vi "FGV_PSP - Mercury Remote.vi"(4 "error in":errorcluster, 6 "Function":enum16{"write", "read"}(ring), 7 "Remote":bool) -> (0 "error out":errorcluster, 3 "Remote":bool)   [LabVIEW 2016, in "Instrument.OxfordVRM.lvclass"]
uses:
  Instrument.OxfordVRM.lvclass
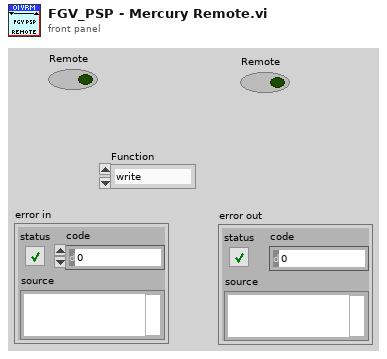
[diagram p1: front panel]
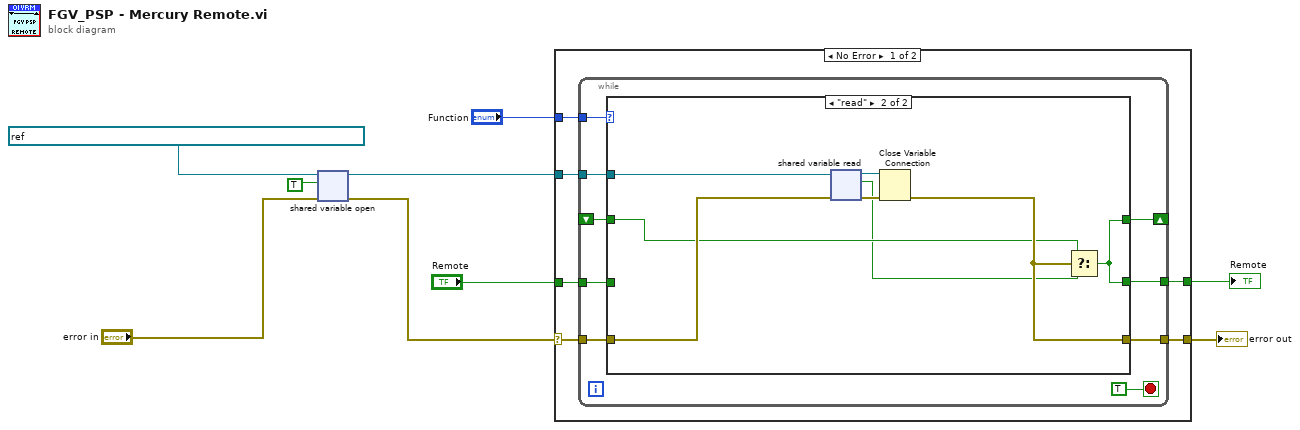
[diagram p0: block diagram]
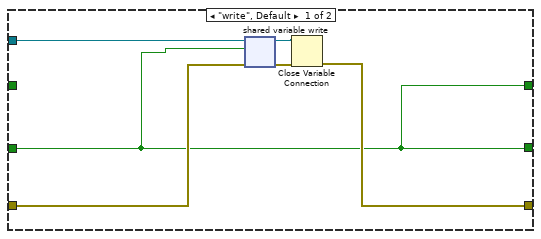
[diagram p2: hidden frame]
diagram:
  n1 = shared-variable-open(refnum<k21> "ni.var.psp://localhost/1820/Mercury_Remote" ("shared variable refnum in"), "error in", TRUE) -> (w7:refnum<k21>, w6:errorcluster)  [unwired: 1 in]
  n2 = case shown="No Error" w6 {
    selector: w6 -> [w15 w40]
    tunnel: [w14 w40] -> w9
    tunnel: [w13 w39] -> w1
    tunnel: "Function" -> [w12 _]
    tunnel: w7 -> [w11 _]
    tunnel: "Remote" -> [w10 w39]
    frame No Error {
      n3 = while {
        shift-right: [w19] -> _
        shift-left: _ -> [w18]
        tunnel: w15 -> [w23]
        tunnel: [w22] -> w14
        tunnel: [w21] -> w13
        tunnel: w12 -> [w20]
        tunnel: w11 -> [w17]
        tunnel: w10 -> [w16]
        stop <- TRUE stop-if-true
        n4 = case shown="\"read\"" w20 {
          tunnel: w23 -> [w29 w36]
          tunnel: [w30 w35] -> w22
          tunnel: [w25 w38] -> w21
          tunnel: [w25 w38] -> w19
          tunnel: w18 -> [_ w34]
          tunnel: w17 -> [w28 w37]
          tunnel: w16 -> [w25 _]
          frame "write", Default {
            n5 = shared-variable-write(w28, w29, w25) -> (w26:refnum<k21>, w27:errorcluster)
            n6 = Close Variable Connection(8:w27, 11:w26) -> (0:w30:errorcluster)
          }
          frame "read" {
            n7 = shared-variable-read(w37, w36) -> (w33:refnum<k21>, w32:errorcluster, w31:bool)  [unwired: 1 out]
            n8 = Close Variable Connection(8:w32, 11:w33) -> (0:w35:errorcluster)
            n9 = Select(t=w34, s=w35, f=w31) -> (s? t:f=w38:bool)
          }
        }
      }
    }
    frame Error {
    }
  }
  "error out" <- w9
  "Remote" <- w1
